vi "HA4BC to Total Energy of Humid Air (Watt).vi"(1 "MFRHA\nMass Flow Rate of Humid Air (Kg/s)":dbl[unit], 2 "Gas Presure":dbl[unit]=80000.0 min=80000.0 max=120000.0, 3 "Tceg":dbl[unit], 4 "RH":dbl) -> (0 "Total Energy of Humid Air (Watt)":dbl[unit])   [LabVIEW 2018]
panel:
  out "Total Energy of Humid Air (Watt)\nTtEnHA=TtEnWV + TtEnDA":dbl[unit](knob)
  out "Total Energy of Dry Air (Watt)":dbl[unit]
  out "Total Energy of Dry Air (Watt)\nTtEnDA=SEDA*MFRDA":dbl[unit](knob) scale=0.0..3500.0
  out "Humidity of Input Air":dbl(knob) scale=0.0..100.0
  out "Total Energy of Water Vapor (Watt)":dbl[unit]
  out "Total Energy of Water Vapor (Watt)\nTtEnWV=SEWV*MFRWV":dbl[unit](knob)
  out "Temprature Of Input Air\nCentigrade Degree":dbl[unit](slide) scale=0.0..100.0
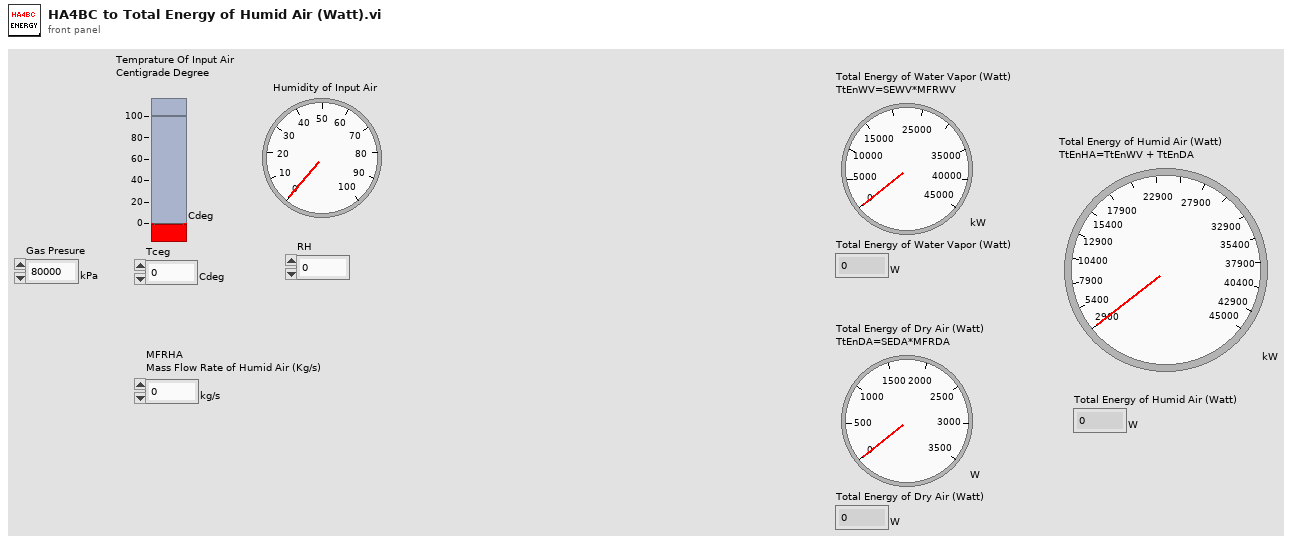
[diagram p1: front panel]
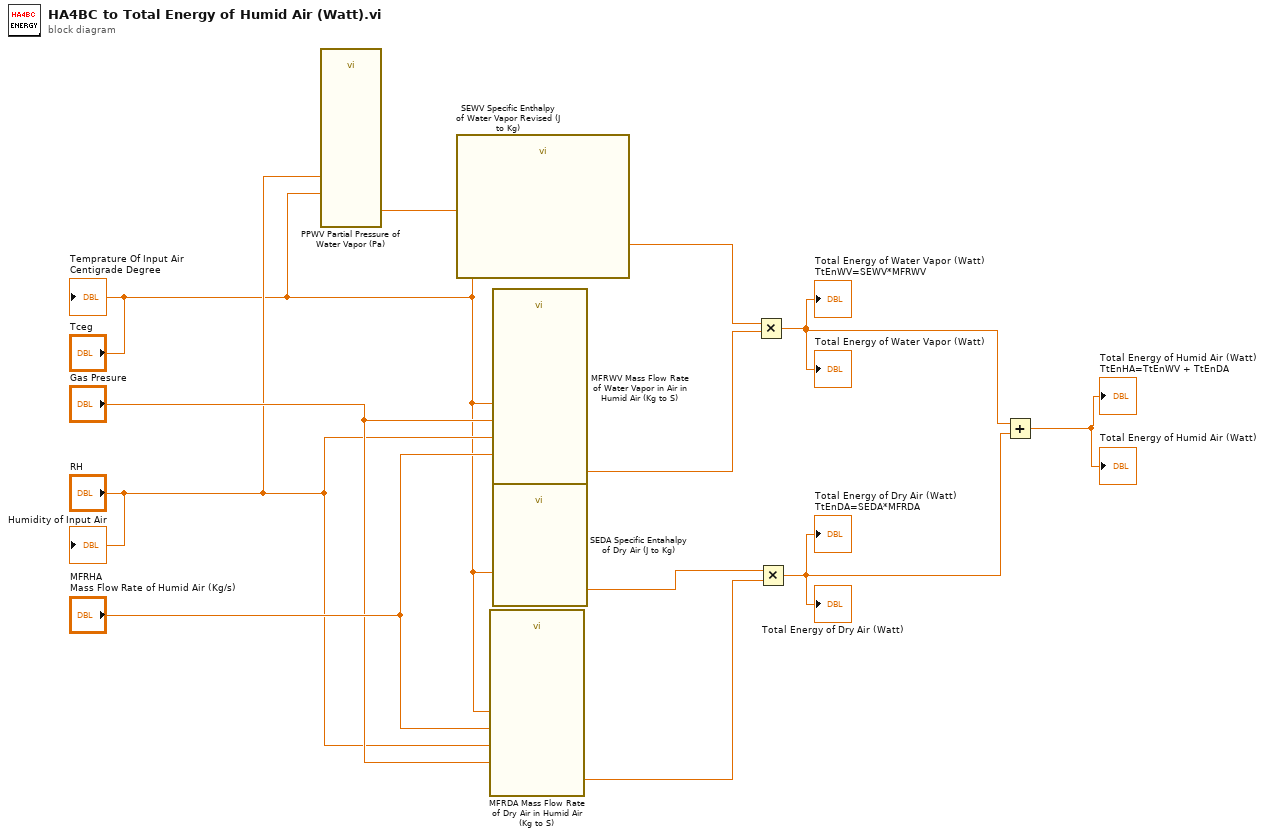
[diagram p0: block diagram]
diagram:
  n1 = call "PPWV Partial Pressure of Water Vapor (Pa).vi"("Tceg"="Tceg", "RH"="RH") -> ("PPWV"=w3:dbl[unit])
  n2 = call "SEWV Specific Enthalpy of Water Vapor Revised (J to Kg).vi"("Partial Pressure of Water Vapor"=w3, "Tceg"="Tceg") -> ("SEWV"=w6:dbl[unit])  [unwired: 1 out]
  n3 = call "MFRDA Mass Flow Rate of Dry Air in Humid Air (Kg to S).vi"("Gas Presure"="Gas Presure", "Tceg"="Tceg", "MFRHA\nMass Flow Rate of Humid Air (Kg/s)"="MFRHA\nMass Flow Rate of Humid Air (Kg/s)", "RH"="RH") -> ("MFRDA"=w11:dbl[unit])
  n4 = call "MFRWV Mass Flow Rate of Water Vapor in Air in Humid Air (Kg to S).vi"("Gas Presure"="Gas Presure", "Tceg"="Tceg", "MFRHA\nMass Flow Rate of Humid Air (Kg/s)"="MFRHA\nMass Flow Rate of Humid Air (Kg/s)", "RH"="RH") -> ("MFRWV"=w4:dbl[unit])
  n5 = call "SEDA Specific Entahalpy of Dry Air (J to Kg).vi"("Tceg"="Tceg") -> ("SEDA"=w12:dbl[unit])
  n6 = Multiply(x=w6, y=w4) -> (x*y=w8:dbl[unit])
  "Total Energy of Water Vapor (Watt)\nTtEnWV=SEWV*MFRWV" <- w8
  "Total Energy of Water Vapor (Watt)" <- w8
  n7 = Multiply(x=w12, y=w11) -> (x*y=w7:dbl[unit])
  "Total Energy of Dry Air (Watt)\nTtEnDA=SEDA*MFRDA" <- w7
  "Total Energy of Dry Air (Watt)" <- w7
  n8 = Add(x=w8, y=w7) -> (x+y=→"Total Energy of Humid Air (Watt)\nTtEnHA=TtEnWV + TtEnDA" →"Total Energy of Humid Air (Watt)":dbl[unit])
  "Temprature Of Input Air\nCentigrade Degree" <- "Tceg"
  "Humidity of Input Air" <- "RH"
